vi "Main Dialog.vi"(11 "Process Path":path) -> ()   [LabVIEW 2020, in "Method Generation.lvlib" / "New Setter Dialog.lvclass"]
uses:
  New Setter Dialog.lvclass
  Setter Generator/Setter Generator.lvclass
panel:
  in  "Highlight changes?":bool=TRUE
  in  "Commit":bool
  in  "Cancel":bool
  in  "Data members":i32(listbox)
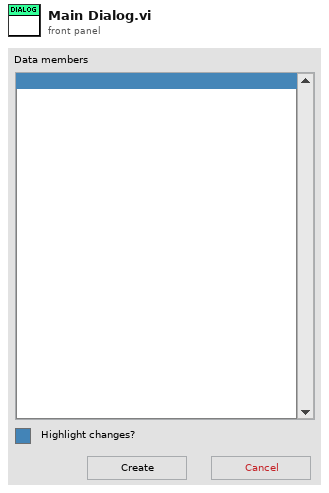
[diagram p1: front panel]
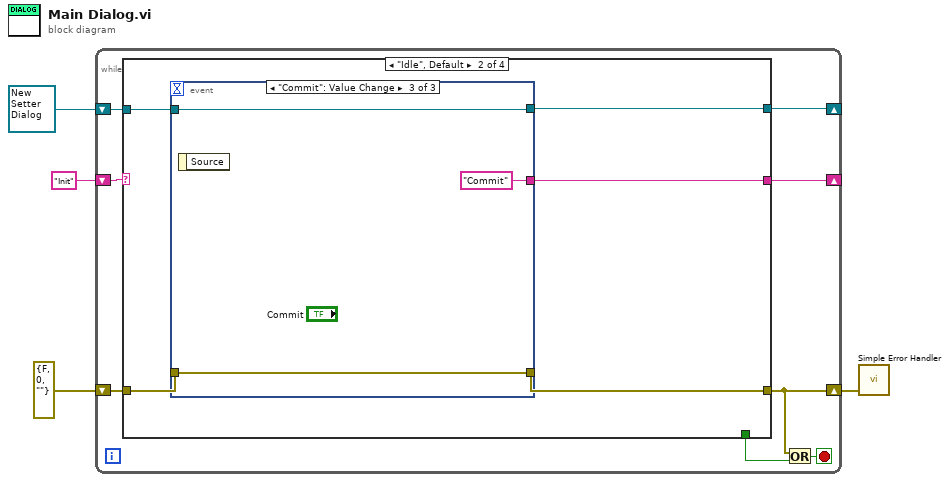
[diagram p0: block diagram]
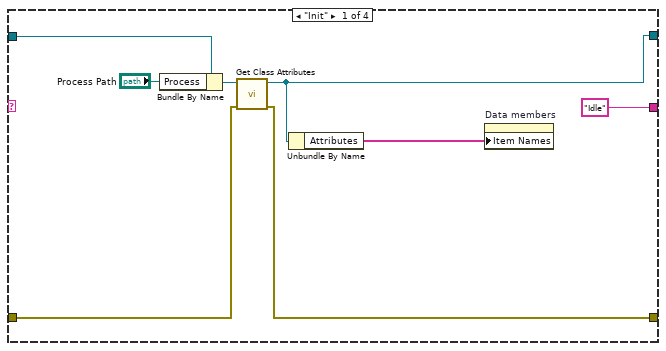
[diagram p2: hidden frame]
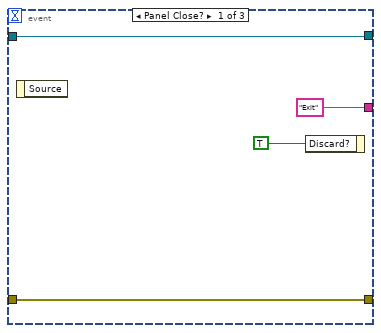
[diagram p3: hidden frame]
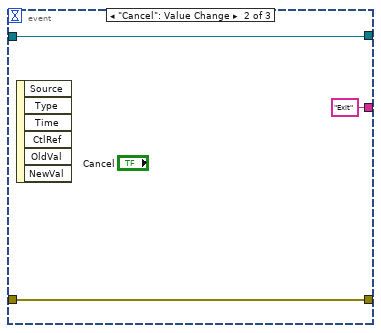
[diagram p4: hidden frame]
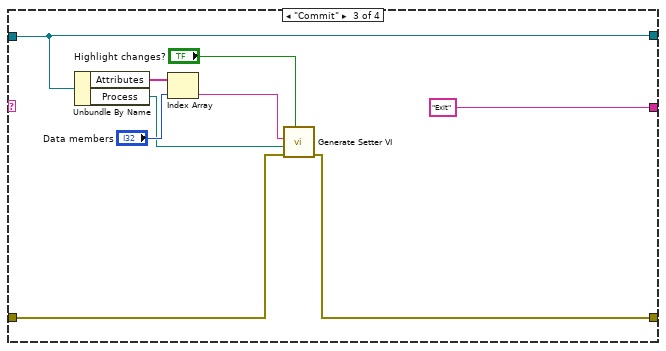
[diagram p5: hidden frame]
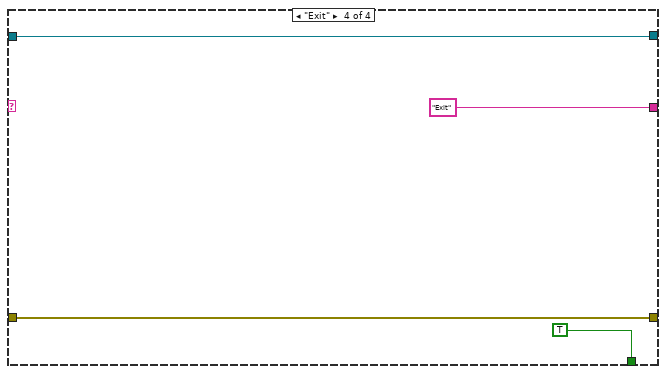
[diagram p6: hidden frame]
diagram:
  n1 = while {
    shift-right: [w9] -> _
    shift-left: refnum<class "New Setter Dialog.lvclass"> refnum ("Method Generation.lvlib:New Getter Dialog.lvclass") -> [w10]
    shift-right: [w5] -> w1
    shift-left: errorcluster {"status"=FALSE, "code"=0, "source"=""} ("error in (no error)") -> [w11]
    shift-right: [w8] -> _
    shift-left: "Init" -> [w12]
    stop <- w6 stop-if-true
    n2 = case shown="\"Idle\", Default" w12 {
      tunnel: [w16 w25 w38 w47] -> w5
      tunnel: w11 -> [w15 w24 w37 w47]
      tunnel: w10 -> [w20 w23 w43 w48]
      tunnel: [w14 w22 w43 w48] -> w9
      tunnel: ["Idle" w21 "Exit" "Exit"] -> w8
      tunnel: [_ _ _ TRUE] -> w7
      frame "Init" {
        n3 = Bundle By Name(cluster=w20, "Process"="Process Path") -> (w17:refnum<class "New Setter Dialog.lvclass">)
        n4 = call "Get Class Attributes.vi"("error in (no error)"=w15, "New Getter Dialog In"=w17) -> ("error out"=w16:errorcluster, "New Getter Dialog Out"=w14:refnum<class "New Setter Dialog.lvclass">)  [unwired: 8 in]
        n5 = Unbundle By Name(w14) -> ("Attributes"=w13:string[])
        n6 = property on="Data members" class="LstBox (strict)"("Item Names"=w13) -> ()  [unwired: 2 in, 2 out]
      }
      frame "Idle", Default {
        n7 = event shown="[2] \"Commit\": Value Change" {
          selector: _ -> [_ _ _]
          dyn-events: _ -> [_ _ _]
          timeout: _ -> [_ _ _]
          tunnel: [w29 w31 w35] -> w25
          tunnel: w24 -> [w29 w31 w35]
          tunnel: w23 -> [w28 w32 w34]
          tunnel: [w28 w32 w34] -> w22
          tunnel: ["Exit" "Exit" "Commit"] -> w21
          event Panel Close? {
            n8 = event-data() -> ()  [unwired: 1 in, 1 out]
            n9 = event-data("Discard?"=TRUE) -> ()  [unwired: 1 in, 1 out]
          }
          event "Cancel": Value Change {
            n10 = event-data() -> ()  [unwired: 1 in, 6 out]
          }
          event "Commit": Value Change {
            n11 = event-data() -> ()  [unwired: 1 in, 1 out]
          }
        }
      }
      frame "Commit" {
        n12 = Unbundle By Name(w43) -> ("Attributes"=w42:string[], "Process"=w39:path)
        n13 = Index Array(array=w42, index="Data members") -> (element=w40:string)
        n14 = call "Generate Setter VI.vi"("Highlight changes?"="Highlight changes?", "error in (no error)"=w37, "class path"=w39, "Attribute Name"=w40) -> ("error out"=w38:errorcluster)  [unwired: 7 in]
      }
      frame "Exit" {
      }
    }
    n15 = Or(x=w5, y=w7) -> (x .or. y?=w6:bool)
  }
  n16 = call <vilib>:"Simple Error Handler.vi"("error in (no error)"=w1) -> ()  [unwired: 4 in, 5 out]
